vi "Set Shooter.vi"(8 "error in":errorcluster, 9 "Feed":dbl, 10 "Rear":dbl, 11 "Front":dbl) -> (0 "error out":errorcluster)   [LabVIEW 2016]
uses:
  Shooterqueue.ctl
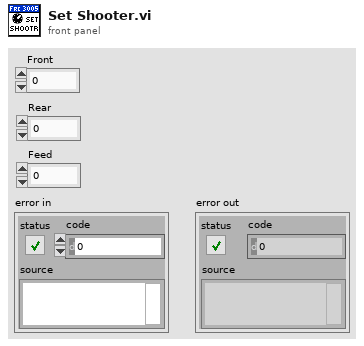
[diagram p1: front panel]
types:
  T1 = typedef "Shooterqueue.ctl" = cluster{"msg":string, "value":dbl}
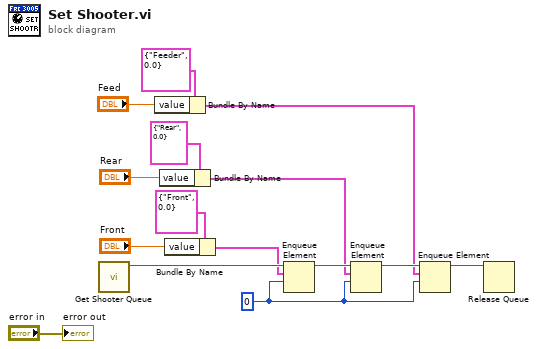
[diagram p0: block diagram]
diagram:
  w1 = 0 ("timeout in ms (-1)")
  n1 = call "Get Shooter Queue.vi"() -> ("Queue out"=w14:refnum<queue>)  [unwired: 10 in, 1 out]
  n2 = Bundle By Name(cluster=T1 {"msg"="Feeder", "value"=0.0} ("Cluster"), "value"="Feed") -> (w3:T1)
  n3 = Bundle By Name(cluster=T1 {"msg"="Rear", "value"=0.0} ("Cluster"), "value"="Rear") -> (w6:T1)
  n4 = Bundle By Name(cluster=T1 {"msg"="Front", "value"=0.0} ("Cluster"), "value"="Front") -> (w12:T1)
  n5 = Enqueue Element(queue=w14, element=w12, timeout in ms (-1)=w1) -> (queue out=w11:refnum<queue>)  [unwired: 1 in, 2 out]
  n6 = Enqueue Element(queue=w11, element=w6, timeout in ms (-1)=w1) -> (queue out=w10:refnum<queue>)  [unwired: 1 in, 2 out]
  n7 = Enqueue Element(queue=w10, element=w3, timeout in ms (-1)=w1) -> (queue out=w2:refnum<queue>)  [unwired: 1 in, 2 out]
  n8 = Release Queue(queue=w2) -> ()  [unwired: 2 in, 3 out]
  "error out" <- "error in"
